vi "BarbHeight.vi"(0 "Refnum in":T2, 1 "ROI Descriptor":T1 {"Contours"."Type" items=["No Selection", "Point", "Line", "Rectangle", "Oval", "Polygon", "Freehand Region", "Annulus", "Unused2", "Unused3", "Broken Line", "Freehand Line", "Rotated Rectangle"]}, 2 "Step Size":u32, 3 "Scan Direction":u16, 4 "Process":T3(ring), 5 "error in (no error)":errorcluster, 6 "Refnum in":T2, 7 "ROI Descriptor 2":T1 {"Contours"."Type" items=["No Selection", "Point", "Line", "Rectangle", "Oval", "Polygon", "Freehand Region", "Annulus", "Unused2", "Unused3", "Broken Line", "Freehand Line", "Rotated Rectangle"]}, 8 "Edge Options":T4 {"Edge Polarity" items=["All Edges", "Rising Edges", "Falling Edges"]; "Minimum Edge Strength" format="%.2f"; "Width" step=2; "Kernel Size" step=2}, 9 "Ta (Constant)":dbl, 10 "AvgMinMax":enum16{"Average", "Max", "Min"}(ring)) -> (14 "Numeric":dbl, 15 "Array":cluster{"X":sgl, "Y":sgl}[](array[cluster]), 16 "a":sgl, 17 "b":sgl, 18 "NumberOfIternations 2":i32, 19 "error out":errorcluster)   [LabVIEW 2019, in "Algorithm.lvclass"]
uses:
  FrameworkOverrides/Algorithm.lvclass
  <vilib>/vision/NI_Vision_Development_Module.lvlib
  <vilib>/vision/Measure.llb/Edge Polarity.ctl
  <vilib>/vision/Measure.llb/Edge Options.ctl
  <vilib>/vision/Image Controls.llb/IMAQ Image.ctl
panel:
  out "Numeric 3":i32
  out "Numeric 2":i32
  out "arccos(x)":sgl
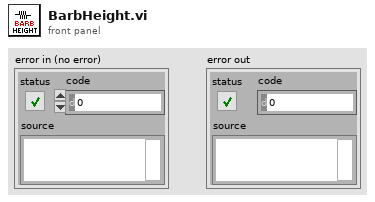
[diagram p1: front panel]
types:
  T1 = typedef "ROI Descriptor" = cluster{"Global Rectangle":i32[], "Contours":cluster{"ID":enum32{"External", "Internal"}, "Type":u32, "Coordinates":i32[]}[]}
  T2 = typedef "IMAQ Image.ctl" = refnum<image>
  T3 = enum16{"Get First Edge", "Get First + Last Edge", "Get All Edges", "Get Best Edge"}
  T4 = typedef "Edge Options.ctl" = cluster{"Edge Polarity":T5, "Kernel Size":u32, "Width":u32, "Minimum Edge Strength":sgl, "Interpolation Type":enum32{"Zero Order", "Bilinear", "Quadratic", "Cubic", "Bilinear Fixed"}, "Data Processing Method":enum32{"Average", "Median"}}
  T5 = typedef "Edge Polarity.ctl" = u32
  T6 = typedef "Edge New.ctl" = cluster{"Location (Pixel)":cluster{"X":sgl, "Y":sgl}, "Location (Real-World)":cluster{"X":sgl, "Y":sgl}, "Distance (Pixel)":dbl, "Distance (Real-World)":dbl, "Strength":dbl, "Noise":dbl, "Rising?":bool}
  T7 = typedef "Search Line.ctl" = cluster{"Start Point":cluster{"X":sgl, "Y":sgl}, "End Point":cluster{"X":sgl, "Y":sgl}, "Edge Info":T6[], "Edge Map":dbl[], "Calibration Valid":bool}
  T8 = cluster{"Real World Coordinates":cluster{"X":sgl, "Y":sgl}, "Real World Coordinates":cluster{"X":sgl, "Y":sgl}}
  T9 = cluster{"Center":cluster{"X":sgl, "Y":sgl}, "Major Axis":cluster{"Point 1":cluster{"X":sgl, "Y":sgl}, "Point 2":cluster{"X":sgl, "Y":sgl}}, "Minor Axis":cluster{"Point 1":cluster{"X":sgl, "Y":sgl}, "Point 2":cluster{"X":sgl, "Y":sgl}}}
  T10 = cluster{"Point 1":cluster{"X":sgl, "Y":sgl}, "Point 2":cluster{"X":sgl, "Y":sgl}, "Point 1":cluster{"X":sgl, "Y":sgl}, "Point 2":cluster{"X":sgl, "Y":sgl}}
  T11 = cluster{"Point 1":cluster{"X":sgl, "Y":sgl}, "Point 1":cluster{"X":sgl, "Y":sgl}}
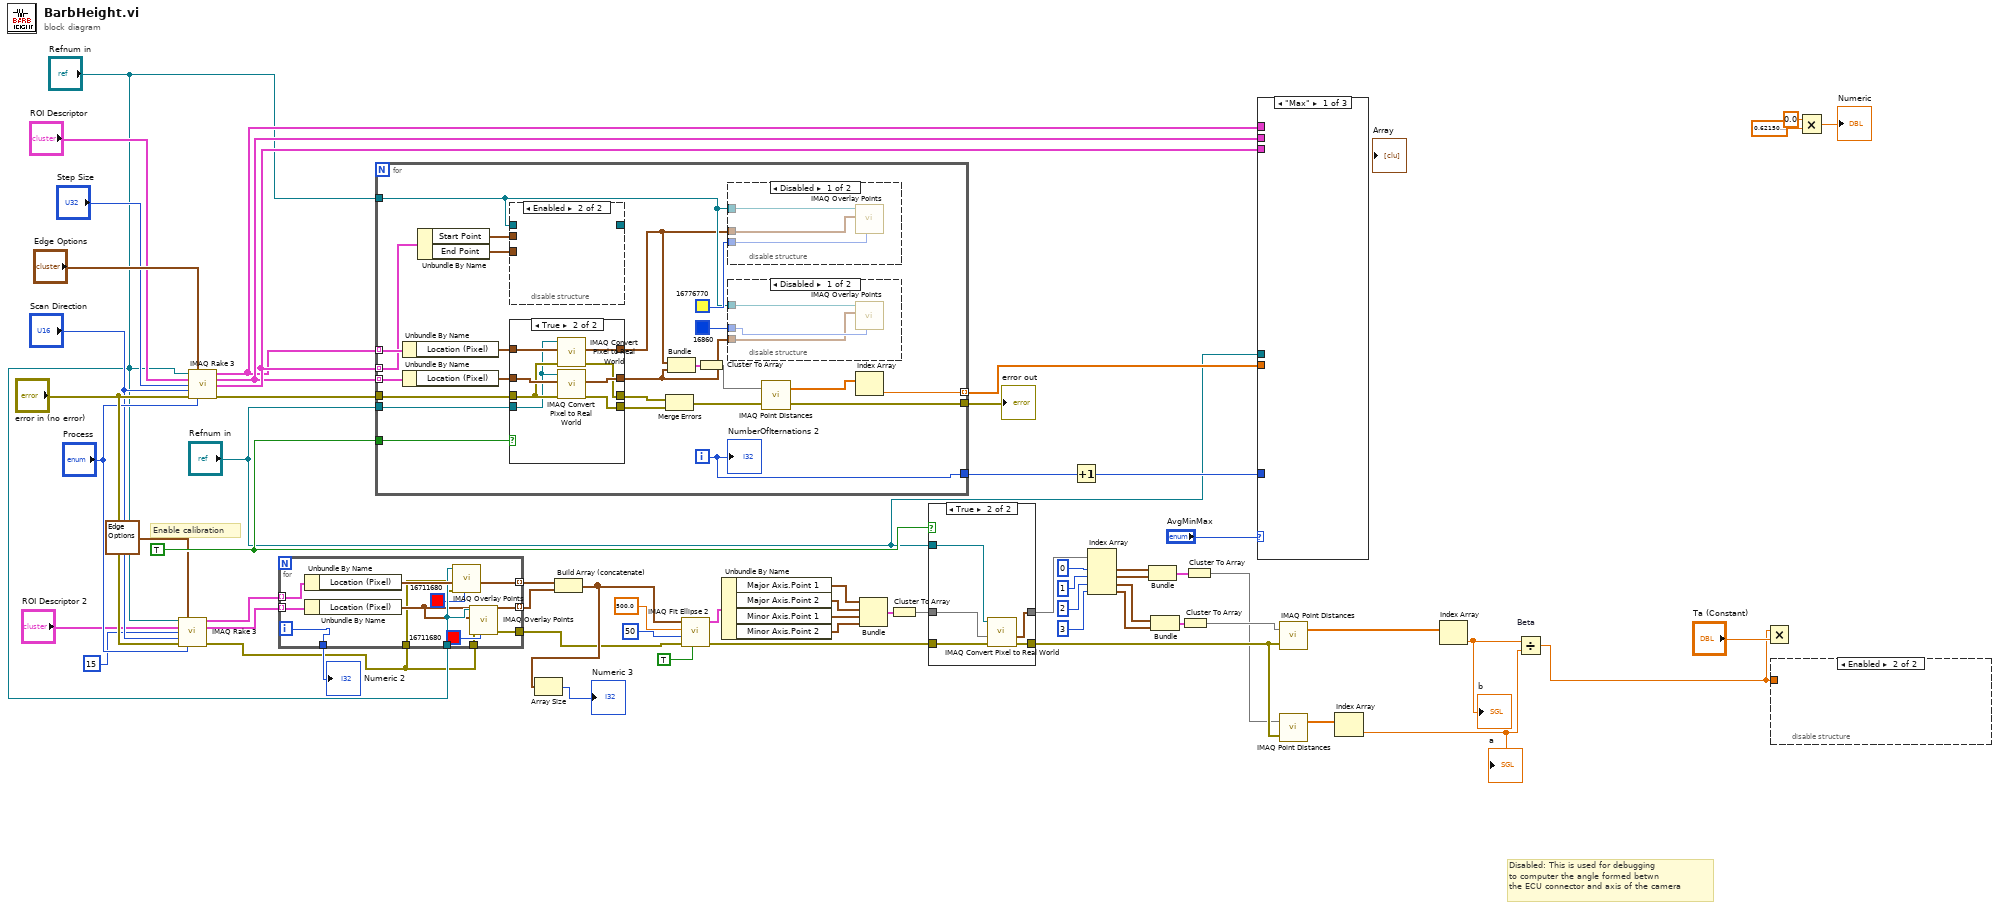
[diagram p0: block diagram]
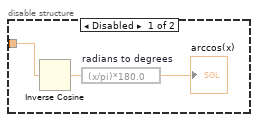
[diagram p2: hidden frame]
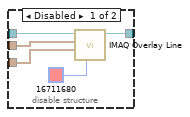
[diagram p9: hidden frame]
diagram:
  w28 = TRUE
  # "Disabled: This is used for debugging\nto computer the angle formed betwn\nthe ECU connector and axis of the camera"
  # "Enable calibration"
  n1 = call "IMAQ Rake 3"("Image"="Refnum in", "Edge Options"=T4 {"Edge Polarity"=0, "Kernel Size"=3, "Width"=3, "Minimum Edge Strength"=50.0, "Interpolation Type"=enum."Zero Order", "Data Processing Method"=enum."Average"}, "ROI Descriptor"="ROI Descriptor 2", "Step Size"=u32 15, "Scan Direction"="Scan Direction", "error in (no error)"="error in (no error)", "Process"="Process") -> ("First Edges"=w48:T6[], "Last Edges"=w49:T6[], "error out"=w16:errorcluster)  [unwired: 5 in, 1 out]
  n2 = call "IMAQ Rake 3"("Image"="Refnum in", "Edge Options"="Edge Options", "ROI Descriptor"="ROI Descriptor", "Step Size"="Step Size", "Scan Direction"="Scan Direction", "error in (no error)"="error in (no error)", "Process"="Process") -> ("First Edges"=w40:T6[], "Last Edges"=w41:T6[], "Search Lines"=w42:T7[], "error out"=w38:errorcluster)  [unwired: 5 in]
  n3 = for {
    tunnel: w48 -> [w75] mode=indexing
    tunnel: w49 -> [w74] mode=indexing
    tunnel: [w73] -> w50 mode=indexing
    tunnel: [w70] -> w51 mode=indexing
    tunnel: [w72] -> w23
    tunnel: "Refnum in" -> [w71]
    tunnel: w16 -> [w67]
    tunnel: w16 -> [w66]
    tunnel: [w65] -> w15
    i -> [w72]
    n4 = Unbundle By Name(w75) -> ("Location (Pixel)"=w73:cluster{"X":sgl, "Y":sgl})
    n5 = Unbundle By Name(w74) -> ("Location (Pixel)"=w70:cluster{"X":sgl, "Y":sgl})
    n6 = call "IMAQ Overlay Points"("Color"=u32 16711680, "error in (no error)"=w66, "Image"=w71) -> ()  [unwired: 7 in, 2 out]
    n7 = call "IMAQ Overlay Points"("Color"=u32 16711680, "error in (no error)"=w67, "Point"=w70, "Image"=w71) -> ("error out"=w65:errorcluster)  [unwired: 6 in, 1 out]
  }
  "Numeric 2" <- w23
  n8 = for {
    tunnel: "Refnum in" -> [w89]
    tunnel: w40 -> [w99] mode=indexing
    tunnel: w41 -> [w98] mode=indexing
    tunnel: w42 -> [w97] mode=indexing
    tunnel: [w92] -> w36 mode=indexing
    tunnel: [w93] -> w35
    tunnel: "Refnum in" -> [w86]
    tunnel: w38 -> [w85]
    tunnel: [w81] -> w39
    tunnel: w28 -> [w80]
    i -> [w93]
    n9 = Unbundle By Name(w99) -> ("Location (Pixel)"=w88:cluster{"X":sgl, "Y":sgl})
    n10 = Unbundle By Name(w98) -> ("Location (Pixel)"=w87:cluster{"X":sgl, "Y":sgl})
    n11 = Unbundle By Name(w97) -> ("Start Point"=w96:cluster{"X":sgl, "Y":sgl}, "End Point"=w95:cluster{"X":sgl, "Y":sgl})
    n12 = disable-structure shown="Enabled" {
      disable-tunnel: w96 -> [w121 _]
      disable-tunnel: w95 -> [w120 _]
      disable-tunnel: w89 -> [w119 _]
      disable-tunnel: [w118 _] -> _
      frame Disabled {
        n13 = call "IMAQ Overlay Line"("Color"=u32 16711680, "End Point"=w120, "Start Point"=w121, "Image"=w119) -> ("Image Out"=w118:T2)  [unwired: 6 in, 1 out]
      }
      frame Enabled {
      }
    }
    n14 = case shown="True" w80 {
      tunnel: [w102 w110] -> w79
      tunnel: w88 -> [w102 w109]
      tunnel: w87 -> [w101 w108]
      tunnel: [w101 w107] -> w78
      tunnel: w86 -> [_ w103]
      tunnel: w85 -> [w100 w106]
      tunnel: [w100 w105] -> w84
      tunnel: [w100 w104] -> w83
      frame False {
      }
      frame True {
        n15 = call "IMAQ Convert Pixel to Real World"("error in (no error)"=w106, "Pixel Coordinates"=w109, "Calibrated Image"=w103) -> ("error out"=w105:errorcluster, "Real World Coordinates"=w110:cluster{"X":sgl, "Y":sgl})  [unwired: 3 in, 4 out]
        n16 = call "IMAQ Convert Pixel to Real World"("error in (no error)"=w106, "Pixel Coordinates"=w108, "Calibrated Image"=w103) -> ("error out"=w104:errorcluster, "Real World Coordinates"=w107:cluster{"X":sgl, "Y":sgl})  [unwired: 3 in, 4 out]
      }
    }
    n17 = Merge Errors(w84, w83) -> (w82:errorcluster)
    n18 = Bundle("Real World Coordinates"=w79, "Real World Coordinates"=w78) -> (w77:T8)  [unwired: 1 in]
    n19 = Cluster To Array(cluster=w77) -> (array=w76:cluster{"X":sgl, "Y":sgl}[])
    n20 = disable-structure shown="Disabled" {
      disable-tunnel: u32 16776770 ("Color") -> [w116 _]
      disable-tunnel: w89 -> [w115 _]
      disable-tunnel: w79 -> [w114 _]
      frame Disabled {
        n21 = call "IMAQ Overlay Points"("Color"=w116, "Point"=w114, "Image"=w115) -> ()  [unwired: 7 in, 2 out]
      }
      frame Enabled {
      }
    }
    n22 = disable-structure shown="Disabled" {
      disable-tunnel: u32 16860 ("Color") -> [w113 _]
      disable-tunnel: w89 -> [w112 _]
      disable-tunnel: w78 -> [w111 _]
      frame Disabled {
        n23 = call "IMAQ Overlay Points"("Color"=w113, "Point"=w111, "Image"=w112) -> ()  [unwired: 7 in, 2 out]
      }
      frame Enabled {
      }
    }
    n24 = call "IMAQ Point Distances"("Points"=w76, "error in (no error)"=w82) -> ("Distances"=w94:sgl[], "error out"=w81:errorcluster)  [unwired: 3 in]
    n25 = Index Array(array=w94) -> (element=w92:sgl)  [unwired: 1 in]
    "NumberOfIternations 2" <- w93
  }
  "error out" <- w39
  n26 = Build Array (concatenate)(w50, w51) -> (w21:cluster{"X":sgl, "Y":sgl}[])
  n27 = Array Size(array=w21) -> (size(s)=→"Numeric 3":i32)
  n28 = call "IMAQ Fit Ellipse 2"("Reject Outliers (FALSE)"=TRUE, "error in (no error)"=w15, "Maximum Iterations"=50, "Minimum Score"=500.0, "Radial Points"=w21) -> ("error out"=w30:errorcluster, "Ellipse"=w31:T9)  [unwired: 1 in, 4 out]
  n29 = Unbundle By Name(w31) -> ("Major Axis.Point 1"=w8:cluster{"X":sgl, "Y":sgl}, "Major Axis.Point 2"=w7:cluster{"X":sgl, "Y":sgl}, "Minor Axis.Point 1"=w6:cluster{"X":sgl, "Y":sgl}, "Minor Axis.Point 2"=w5:cluster{"X":sgl, "Y":sgl})
  n30 = Bundle("Point 1"=w8, "Point 2"=w7, "Point 1"=w6, "Point 2"=w5) -> (w4:T10)  [unwired: 1 in]
  n31 = Cluster To Array(cluster=w4) -> (array=w3:cluster{"X":sgl, "Y":sgl}[])
  n32 = case shown="True" w28 {
    tunnel: [w122 w128] -> w60
    tunnel: [w123 w127] -> w55
    tunnel: w3 -> [w123 w126]
    tunnel: w30 -> [w122 w125]
    tunnel: "Refnum in" -> [_ w124]
    frame False {
    }
    frame True {
      n33 = call "IMAQ Convert Pixel to Real World"("error in (no error)"=w125, "Array of Pixel Coordinates"=w126, "Calibrated Image"=w124) -> ("error out"=w128:errorcluster, "Array of Real World Coordinates"=w127:cluster{"X":sgl, "Y":sgl}[])  [unwired: 3 in, 4 out]
    }
  }
  n34 = Increment(x=w35) -> (x+1=w34:i32)
  n35 = Index Array(array=w55, index #1=0 ("index"), index #2=1 ("index"), index #3=2 ("index"), index #4=3 ("index")) -> (element #1=w14:cluster{"X":sgl, "Y":sgl}, element #2=w13:cluster{"X":sgl, "Y":sgl}, element #3=w11:cluster{"X":sgl, "Y":sgl}, element #4=w10:cluster{"X":sgl, "Y":sgl})
  n36 = Bundle("Point 1"=w14, "Point 1"=w13) -> (w12:T11)  [unwired: 1 in]
  n37 = Bundle("Point 1"=w11, "Point 1"=w10) -> (w9:T11)  [unwired: 1 in]
  n38 = Cluster To Array(cluster=w9) -> (array=w2:cluster{"X":sgl, "Y":sgl}[])
  n39 = Cluster To Array(cluster=w12) -> (array=w1:cluster{"X":sgl, "Y":sgl}[])
  n40 = case shown="\"Max\"" "AvgMinMax" {
    tunnel: w34 -> [_ _ _]
    tunnel: w36 -> [_ _ _]
    tunnel: w40 -> [_ _ _]
    tunnel: w41 -> [_ _ _]
    tunnel: w42 -> [_ _ _]
    tunnel: "Refnum in" -> [_ _ _]
    frame "Max" {
    }
    frame "Min" {
    }
    frame "Average" {
    }
  }
  n41 = call "IMAQ Point Distances"("Points"=w2, "error in (no error)"=w60) -> ("Distances"=w62:sgl[])  [unwired: 3 in, 1 out]
  n42 = call "IMAQ Point Distances"("Points"=w1, "error in (no error)"=w60) -> ("Distances"=w61:sgl[])  [unwired: 3 in, 1 out]
  n43 = Index Array(array=w61) -> (element=w25:sgl)  [unwired: 1 in]
  "a" <- w25
  n44 = Index Array(array=w62) -> (element=w26:sgl)  [unwired: 1 in]
  "b" <- w26
  n45 = Divide "Beta"(x=w26, y=w25) -> (x/y=w24:sgl)
  n46 = Multiply(x=w24, y="Ta (Constant)") -> ()  [unwired: 1 out]
  n47 = disable-structure shown="Enabled" {
    disable-tunnel: w24 -> [w131 _]
    frame Disabled {
      n48 = Inverse Cosine(1:w131) -> (0:w130:sgl)
      n49 = expression code="(x/pi)*180.0" "radians to degrees"(w130) -> (→"arccos(x)":sgl)
    }
    frame Enabled {
    }
  }
  n50 = Multiply(x=sgl 0.0, y=sgl 0.6215) -> (x*y=→"Numeric":sgl)
